vi "Get ControlRef from LibraryItem.vi"(8 "error in (no error)":errorcluster, 10 "Control Name":string, 11 "Library item in":refnum<vi>) -> (0 "error out":errorcluster, 1 "Found?":bool, 2 "Control ref out":refnum<vi>, 3 "Library item out":refnum<vi>)   [LabVIEW 2019, in "gRPC Scripting Tools.lvlib"]
uses:
  gRPC Scripting Tools.lvlib
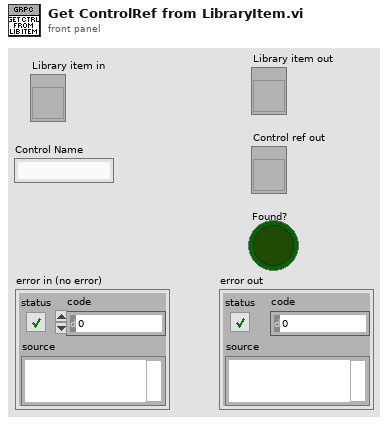
[diagram p1: front panel]
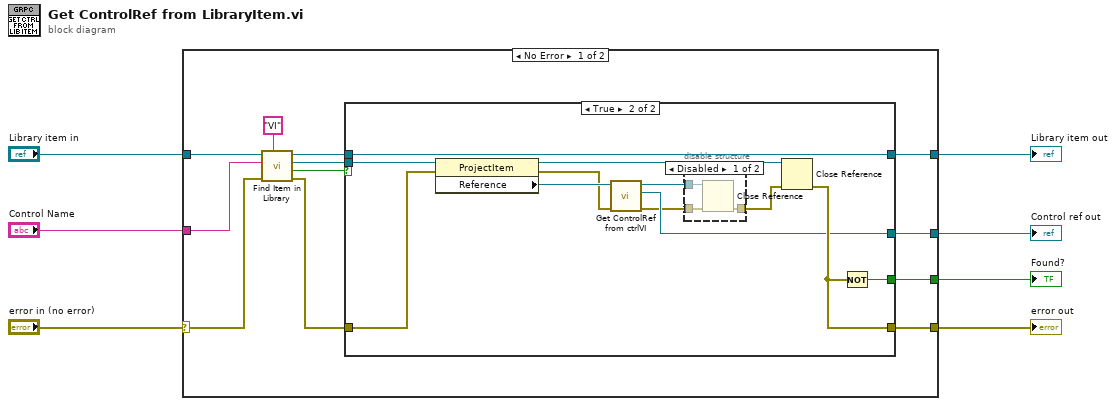
[diagram p0: block diagram]
diagram:
  n1 = case shown="No Error" "error in (no error)" {
    selector: "error in (no error)" -> [w10 w39]
    tunnel: [w19 _] -> w7
    tunnel: [w14 w39] -> w6
    tunnel: "Library item in" -> [w17 w38]
    tunnel: "Control Name" -> [w16 _]
    tunnel: [w11 w38] -> w2
    tunnel: [w8 _] -> w1
    frame No Error {
      n2 = call "Find Item in Library.vi"("Item Type"="VI" ("Type"), "error in (no error)"=w10, "Item Name"=w16, "Library item in"=w17) -> ("error out"=w9:errorcluster, "Found?"=w13:bool, "Project Item (Library Item)"=w15:refnum<vi>, "Library item out"=w12:refnum<vi>)  [unwired: 4 in]
      n3 = case shown="True" w13 {
        tunnel: [_ w25] -> w19
        tunnel: w9 -> [w20 w31]
        tunnel: w15 -> [_ w30]
        tunnel: [w20 w27] -> w14
        tunnel: w12 -> [w21 w28]
        tunnel: [w21 w28] -> w11
        tunnel: [_ w26] -> w8
        frame False {
        }
        frame True {
          n4 = property class="ProjectItem"(reference=w30, error in=w31) -> (reference out=w29:refnum<vi>, error out=w32:errorcluster, "Reference"=w33:refnum<vi>)
          n5 = call "Get ControlRef from ctrlVI.vi"("error in (no error)"=w32, "VI ref in"=w33) -> ("error out"=w23:errorcluster, "Control ref out"=w25:refnum<vi>, "VI ref out"=w24:refnum<vi>)  [unwired: 7 in]
          n6 = disable-structure shown="Disabled" {
            disable-tunnel: w24 -> [w36 _]
            disable-tunnel: w23 -> [w35 w37]
            disable-tunnel: [w34 w37] -> w22
            frame Disabled {
              n7 = Close Reference(reference=w36, error in (no error)=w35) -> (error out=w34:errorcluster)
            }
            frame Enabled {
            }
          }
          n8 = Close Reference(reference=w29, error in (no error)=w22) -> (error out=w27:errorcluster)
          n9 = Not(x=w27) -> (.not. x?=w26:bool)
        }
      }
    }
    frame Error {
    }
  }
  "Control ref out" <- w7
  "error out" <- w6
  "Library item out" <- w2
  "Found?" <- w1
